vi "ULS Z Stack.vi"(8 "error in (no error)":errorcluster, 10 "Z Stack Para(um)":cluster{"Start":dbl, "End":dbl, "Interval":dbl}, 11 "IFD in":refnum<class "IFD.lvclass">) -> (0 "error out":errorcluster, 3 "IFD out":refnum<class "IFD.lvclass">)   [LabVIEW 2016, in "IFD.lvclass"]
uses:
  IFD.lvclass
  Tag/IFD_Tag.lvclass/IFD_Tag.ctl
  IFD.lvclass/IFD.ctl
  Tag/IFD_Tag.lvclass
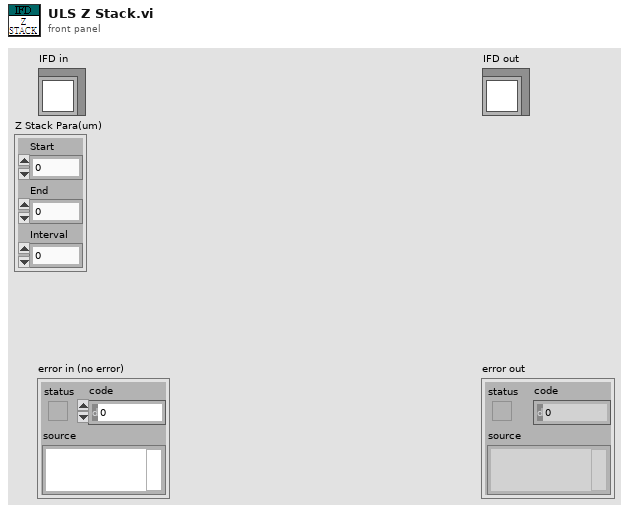
[diagram p1: front panel]
types:
  T1 = enum16{"Undefined(DO NOT USE)", "U8", "ASCII", "U16", "U32", "RATIONAL", "I8", "Undefined 8 bit", "I16", "I32", "SRATIONAL", "SGL", "DBL"}
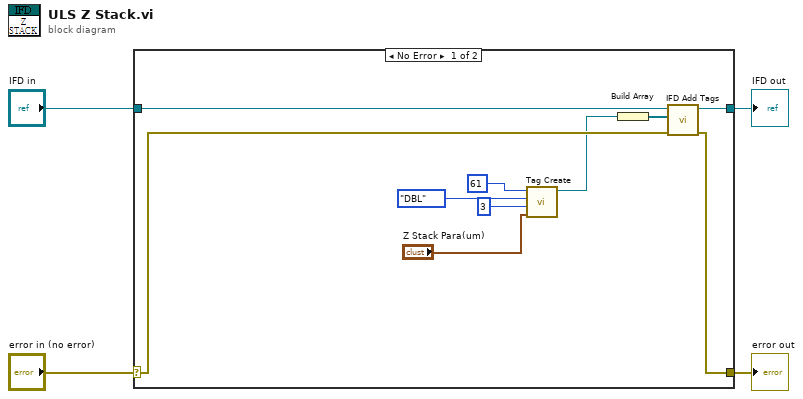
[diagram p0: block diagram]
diagram:
  n1 = case shown="No Error" "error in (no error)" {
    selector: "error in (no error)" -> [w11 w16]
    tunnel: [w10 w16] -> w3
    tunnel: [w13 w15] -> w1
    tunnel: "IFD in" -> [w14 w15]
    frame No Error {
      n2 = call "Tag Create.vi"("Data"="Z Stack Para(um)", "Data Count"=u32 3, "Data Type"=T1."DBL", "Tag ID"=u16 61) -> ("IFD_Tag out"=w9:refnum<class "IFD_Tag.lvclass">)  [unwired: 7 in]
      n3 = Build Array(w9) -> (w12:refnum<class "IFD_Tag.lvclass">[])
      n4 = call "IFD Add Tags.vi"("error in (no error)"=w11, "Tag(s)"=w12, "IFD in"=w14) -> ("error out"=w10:errorcluster, "IFD out"=w13:refnum<class "IFD.lvclass">)  [unwired: 7 in]
    }
    frame Error {
    }
  }
  "error out" <- w3
  "IFD out" <- w1
